vi "Stop Core.vi"(10 "final error code":i32, 11 "Simulated Entry Console Actor in":refnum<class "Simulated Entry Console Actor.lvclass">) -> (3 "Simulated Entry Console Actor out":refnum<class "Simulated Entry Console Actor.lvclass">)   [LabVIEW 2019, in "Simulated Entry Console Actor.lvlib" / "Simulated Entry Console Actor.lvclass"]
doc: "(<B>Filename</B>: Actor Framework.lvlib:Actor.lvclass:Stop Core.vi)\n\nDefines what the actor does before it stops. Use the <B>final error code</B> input to determine whether the actor shut down in response to an error.\n\nBy default, this method passes the Stop message along to all auto-stop nested actors. A descendant class may override this method to define additional behavior, such as shutting down any processes the actor initiated in its override of the Actor Core method."
uses:
  Simulated Entry Console Actor.lvclass
  Simulated Entry Console Actor.lvclass/Simulated Entry Console Actor.ctl
  Abstract Entry Console Actor/Abstract Entry Console Actor/Entry Console Actor.lvclass
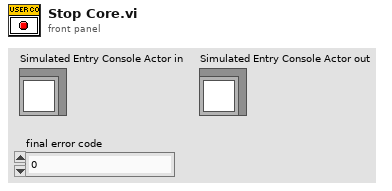
[diagram p1: front panel]
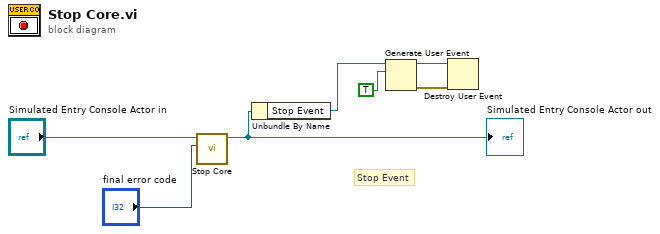
[diagram p0: block diagram]
diagram:
  # "Stop Event"
  n1 = call-parent "Stop Core.vi"("final error code"="final error code", "Actor in"="Simulated Entry Console Actor in") -> ("Actor out"=w3:refnum<class "Simulated Entry Console Actor.lvclass">)  [unwired: 9 in]
  "Simulated Entry Console Actor out" <- w3
  n2 = Unbundle By Name(w3) -> ("Stop Event"=w2:refnum<user-event>)
  n3 = Generate User Event(user event=w2, event data cluster=TRUE ("event data")) -> (user event out=w5:refnum<user-event>, error out=w4:errorcluster)  [unwired: 2 in]
  n4 = Destroy User Event(user event=w5, error in=w4) -> ()  [unwired: 1 out]
